vi "readFromXML.vi"(8 "error in (no error)":errorcluster, 10 "XML in":string, 11 "WSMode in":refnum<class "WSMode.lvclass">) -> (0 "error out":errorcluster, 3 "WSMode out":refnum<class "WSMode.lvclass">)   [LabVIEW 2022 SP3, in "TCSDataDefinitions.lvlib" / "TCSWeatherServerCommand.lvlib" / "WSMode.lvclass"]
uses:
  WSMode.lvclass
  Enumerations/wsMode.ctl
  WSMode.lvclass/WSMode.ctl
  TCSWeatherServerCommand/TCSWeatherServerCommand.lvclass
  <userlib>/Common/XML/XMLParser/XMLParser.lvclass
  TCSWeatherServerCommand.lvlib
panel:
  out "wsMode":T1
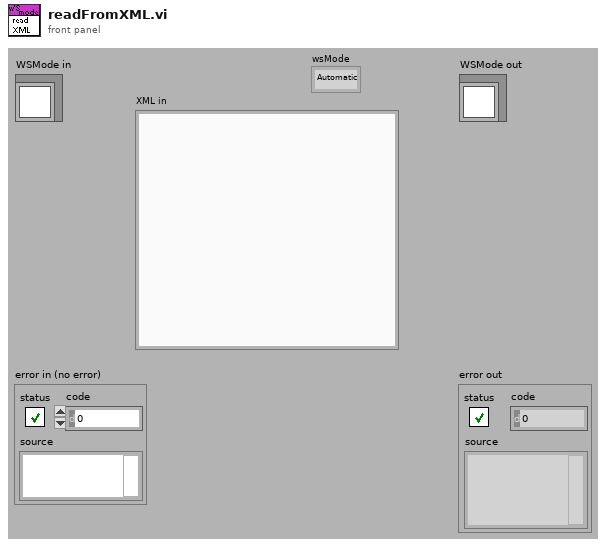
[diagram p1: front panel]
types:
  T1 = typedef "TCSDataDefinitions.lvlib/TCSWeatherServerCommand.lvlib/wsMode.ctl" = enum16{"Automatic", "Manual"}
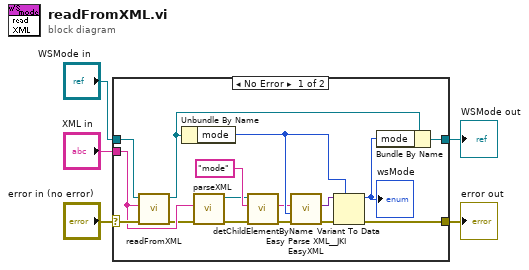
[diagram p0: block diagram]
diagram:
  n1 = case shown="No Error" "error in (no error)" {
    selector: "error in (no error)" -> [w13 w23]
    tunnel: [w14 w23] -> w4
    tunnel: [w17 w22] -> w2
    tunnel: "WSMode in" -> [w16 w22]
    tunnel: "XML in" -> [w8 _]
    frame No Error {
      n2 = call-parent "readFromXML.vi"("error in (no error)"=w13, "XML in"=w8, "TCSWeatherServerCommand in"=w16) -> ("error out"=w7:errorcluster, "TCSWeatherServerCommand out"=w15:refnum<class "WSMode.lvclass">)  [unwired: 7 out]
      n3 = Unbundle By Name(w15) -> ("mode"=w19:T1)
      n4 = call <userlib>:"parseXML.vi"("error in (no error)"=w7, "XMLString in"=w8) -> ("error out"=w12:errorcluster, "Element out"=w6:refnum<class "XMLParser.lvclass">)  [unwired: 8 in]
      n5 = call <userlib>:"detChildElementByName.vi"("error in (no error)"=w12, "childName"="mode" ("ChildName"), "Element in"=w6) -> ("error out"=w9:errorcluster, "childXML"=w10:string)  [unwired: 5 in, 2 out]
      n6 = call <vilib>:"Easy Parse XML__JKI EasyXML.vi"("error in (no error)"=w9, "LabVIEW Data (Type)"=w19, "XML String"=w10) -> ("error out"=w21:errorcluster, "LabVIEW Data"=w20:variant)  [unwired: 7 out]
      n7 = Variant To Data(error in=w21, type=w19, Variant=w20) -> (data=w18:T1, error out=w14:errorcluster)
      "wsMode" <- w18
      n8 = Bundle By Name(cluster=w15, "mode"=w18) -> (w17:refnum<class "WSMode.lvclass">)
    }
    frame Error {
    }
  }
  "error out" <- w4
  "WSMode out" <- w2
